vi "ControlDataSecond.vi"(0 "Numeric":i32=3, 1 "Boolean":bool, 2 "array":string[][](array[string])) -> ()   [LabVIEW 2014]
doc: "This Sub VI accepts a string for units, and a 2D array containing values for data point #, times in seconds and pressure in the units the user inputs before the user pressure the acquire button. This SUB VI, then, saves the data into a CSV file, which is saved in the same location where the main program and this SUB VI is located in."
uses:
  <vilib>/Utility/file.llb/Write To Spreadsheet File (string).vi
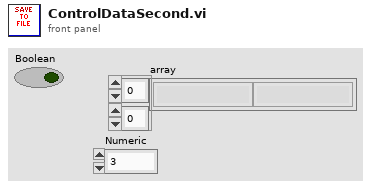
[diagram p1: front panel]
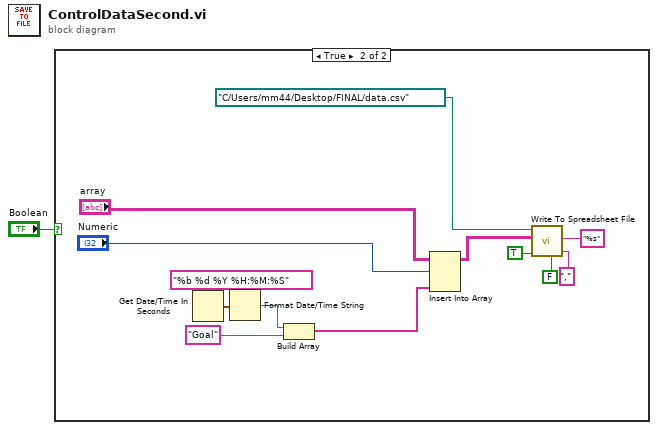
[diagram p0: block diagram]
diagram:
  n1 = case shown="True" "Boolean" {
    frame False {
    }
    frame True {
      n2 = Get Date/Time In Seconds() -> (seconds since 1Jan1904=w8:timestamp)
      n3 = Format Date/Time String(time format string (%c)="%b %d %Y %H:%M:%S", seconds (now)=w8) -> (date/time string=w6:string)  [unwired: 1 in]
      n4 = Build Array(w6, "Goal") -> (w10:string[])
      n5 = Insert Into Array(array="array", index (row)="Numeric", new element=w10) -> (w4:string[][])  [unwired: 1 in]
      n6 = call-poly <vilib>:"Write To Spreadsheet File.vi"("delimiter (\\t)"="," ("delimiter (\\t)"), "transpose? (no:F)"=FALSE ("append to file? (new file:F)"), "format (%s)"="%s" ("format (%.3f)"), "append to file? (new file:F)"=TRUE, "2D data"=w4, "file path (dialog if empty)"=path "C:/Users/mm44/Desktop/FINAL/data.csv" ("Path")) -> ()  [unwired: 2 in, 1 out]
    }
  }
